vi "Main.vi"() -> ()   [LabVIEW 2018]
panel:
  out "R_max":dbl
  out "R_min":dbl
  in  "format string":string
  out "match substring":string
  in  "regular expression":string
  out "text":string
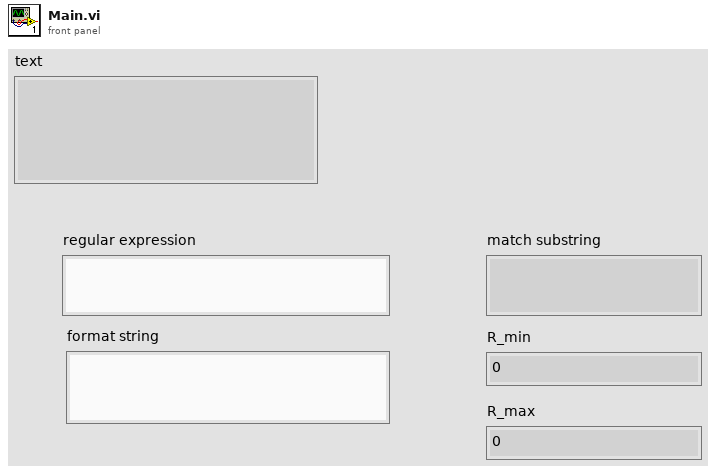
[diagram p1: front panel]
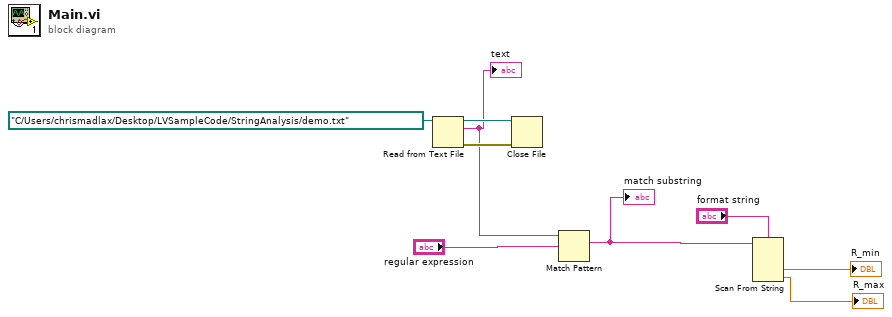
[diagram p0: block diagram]
diagram:
  n1 = Read from Text File(file (use dialog)=path "C:/Users/chrismadlax/Desktop/LVSampleCode/StringAnalysis/demo.txt") -> (refnum out=w9:refnum<file>, text=w6:string, error out=w8:errorcluster)  [unwired: 3 in, 1 out]
  "text" <- w6
  n2 = Close File(refnum=w9, error in=w8) -> ()  [unwired: 2 out]
  n3 = Match Pattern(string=w6, regular expression="regular expression") -> (match substring=w4:string)  [unwired: 1 in, 3 out]
  "match substring" <- w4
  n4 = Scan From String(format string="format string", input string=w4) -> (output 1=→"R_min":dbl, output 2=→"R_max":dbl)  [unwired: 4 in, 3 out]
